vi "databaseTesting.vi"() -> ()   [LabVIEW 2017]
doc: "Use this template to build a VI to use as a subVI."
uses:
  <vilib>/addons/Database/Connection.llb/DB Tools Open Connec (Path).vi
  <vilib>/addons/Database/NI_Database_API.lvlib
panel:
  out "Image":T1(plugin-control)
  in  "File Path":path=path "C:/Users/OmerLab/Documents/GitHub/RamanSpecUsingStageXY/imagesForTesting/Snap-15.jpg"
  out "Core Pressure":dbl[](graph)
  out "Core Temperature":dbl[](graph)
  out "max pressure value":dbl format="%#.6g"
  out "min pressure value":dbl format="%#.6g"
  out "max temperature value":dbl format="%#.6g"
  out "min temperature value":dbl format="%#.6g"
  in  "Stop":bool
  out "Number of Records":i32
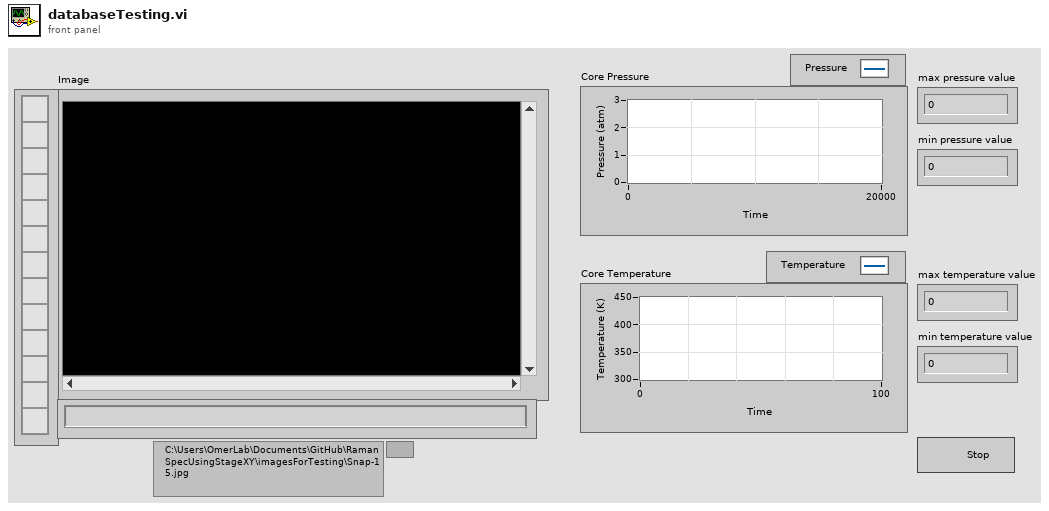
[diagram p1: front panel]
types:
  T1 = typedef "IMAQ Image.ctl" = refnum<image>
  T2 = typedef "Image Type" = u32
  T3 = typedef "NI_Database_API.lvlib/Conn ObjectReference.ctl" = refnum<k1>
  T4 = cluster{i32, string, dbl, dbl, "FileString":string, dbl, dbl}
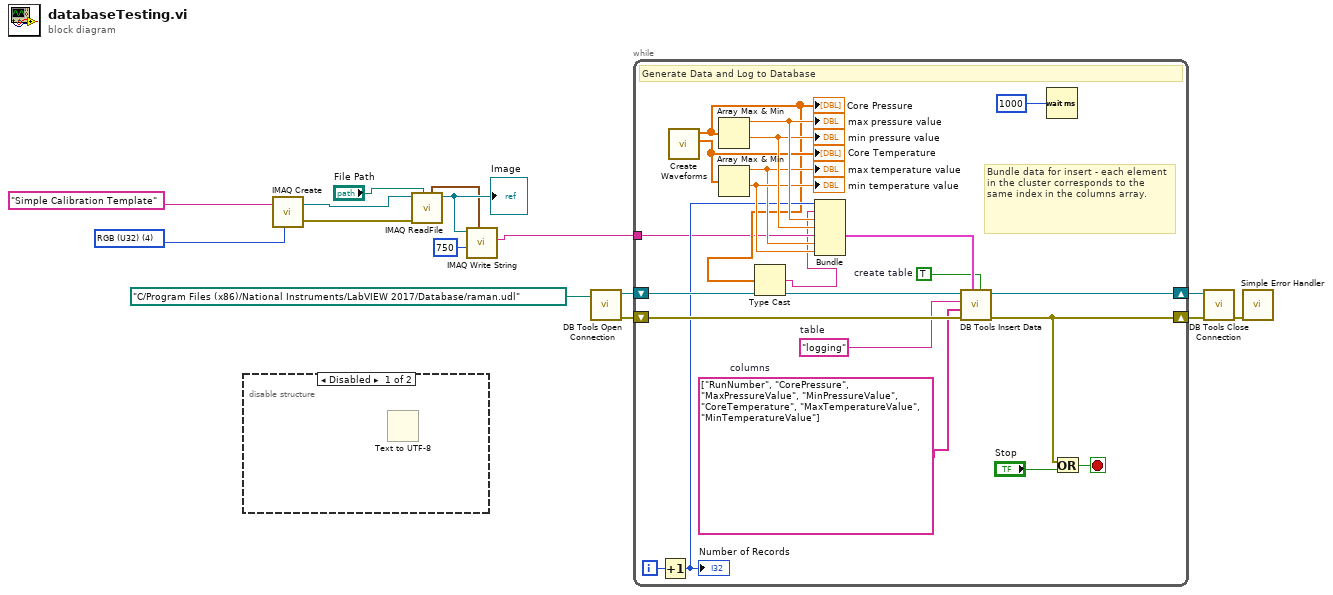
[diagram p0: block diagram]
diagram:
  w6 = T2 4 items=["Grayscale (U8)", "Grayscale (I16)", "Grayscale (SGL)", "Complex (CSG)", "RGB (U32)", "HSL (U32)", "RGB (U64)", "Grayscale (U16)"] ("Image Type")
  n1 = disable-structure shown="Disabled" {
    frame Disabled {
      n2 = Text to UTF-8() -> ()  [unwired: 3 in, 2 out]
    }
    frame Enabled {
    }
  }
  n3 = call "IMAQ Create"("Image Name"="Simple Calibration Template", "Image Type"=w6) -> ("New Image"=w8:T1, "error out"=w10:errorcluster)  [unwired: 2 in, 1 out]
  n4 = call "IMAQ ReadFile"("File Path"="File Path", "error in (no error)"=w10, "Image"=w8) -> ("Image Out"=w4:T1, "Color Palette out"=w3:cluster{"Red":u8, "Green":u8, "Blue":u8}[])  [unwired: 4 in, 3 out]
  "Image" <- w4
  n5 = call-poly "IMAQ Write String"("Color Palette"=w3, "Image Quality"=u32 750, "Image"=w4) -> ("FileString"=w1:string)  [unwired: 6 in, 2 out]
  n6 = call-poly <vilib>:"DB Tools Open Connection.vi"("connection information"=path "C:/Program Files (x86)/National Instruments/LabVIEW 2017/Database/raman.udl") -> ("error out"=w14:errorcluster, "connection reference"=w15:T3)  [unwired: 7 in]
  n7 = while {
    shift-right: [w21] -> w12
    shift-left: w14 -> [w29]
    shift-right: [w31] -> w13
    shift-left: w15 -> [w30]
    tunnel: w1 -> [w17]
    i -> [w32]
    stop <- w25 stop-if-true
    w19 = string[] ["RunNumber", "CorePressure", "MaxPressureValue", "MinPressureValue", "CoreTemperature", "MaxTemperatureValue", "MinTemperatureValue"]  # columns
    w20 = "logging"  # table
    w27 = TRUE  # create table
    # "Bundle data for insert - each element in the cluster corresponds to the same index in the columns array."
    # "Generate Data and Log to Database"
    n8 = Increment(x=w32) -> (x+1=w23:i32)
    "Number of Records" <- w23
    n9 = call "Create Waveforms.vi"() -> ("core temperature"=w24:dbl[], "core pressure"=w18:dbl[])  [unwired: 10 in]
    "Core Pressure" <- w18
    "Core Temperature" <- w24
    n10 = Array Max & Min(array=w18) -> (max value=w36:dbl, min value=w35:dbl)  [unwired: 2 out]
    "max pressure value" <- w36
    "min pressure value" <- w35
    n11 = Array Max & Min(array=w24) -> (max value=w33:dbl, min value=w34:dbl)  [unwired: 2 out]
    "max temperature value" <- w33
    "min temperature value" <- w34
    n12 = Type Cast(x=w18) -> (*(type *) &x=w16:string)  [unwired: 1 in]
    n13 = Bundle(w23, w16, w36, w35, "FileString"=w17, w33, w34) -> (w28:T4)  [unwired: 1 in]
    n14 = call <vilib>:"DB Tools Insert Data.vi"("create table? (F)"=w27, "data"=w28, "error in (no error)"=w29, "columns"=w19, "table"=w20, "connection reference"=w30) -> ("error out"=w21:errorcluster, "connection reference out"=w31:T3)  [unwired: 4 in]
    n15 = Wait (ms)(milliseconds to wait=u32 1000) -> ()  [unwired: 1 out]
    n16 = Or(x=w21, y="Stop") -> (x .or. y?=w25:bool)
  }
  n17 = call <vilib>:"DB Tools Close Connection.vi"("error in (no error)"=w12, "connection reference"=w13) -> ("error out"=w11:errorcluster)  [unwired: 5 in]
  n18 = call <vilib>:"Simple Error Handler.vi"("error in (no error)"=w11) -> ()  [unwired: 4 in, 5 out]
